vi "PrimaryAttackerRole_v2.vi"(7 "firstCall":bool=TRUE, 8 "error in (no error)":errorcluster, 10 "Game in":refnum<class "Game.lvclass">, 11 "ShootRole in":refnum<class "PrimaryAttackerRole_v2.lvclass">) -> (0 "error out":errorcluster, 1 "Game out":refnum<class "Game.lvclass">, 2 "Robot out":refnum<class "Robot.lvclass">, 3 "ShootRole out":refnum<class "PrimaryAttackerRole_v2.lvclass">)   [LabVIEW 2023, in "PrimaryAttackerRole_v2.lvclass"]
uses:
  PrimaryAttackerRole_v2.lvclass
  C:/Users/ebert/Documents/codes/SSL/repo/SSL_AI/Role_class/Role.lvclass
  Game_class/Game.lvclass
  Robot_class/Robot.lvclass
  Role_class/Role.lvclass/Role.ctl
  PrimaryAttacker_class/PrimaryAttackerRole_states.ctl
  PrimaryAttackerRole_v2.lvclass/PrimaryAttackerRole_v2.ctl
  Robot_class/tactics.ctl
  Robot_class/Robot.lvclass/Robot.ctl
  Tacticbook_class/Tacticbook.lvclass/Tacticbook.ctl
  Tacticbook_class/Read WaitPassTactic.vi
  Robot_class/Write tactic.vi
  Tacticbook_class/Read ShootTactic.vi
  Role_class/Read Tacticbook.vi
  Read Tactics.vi
  Role_class/Write Tacticbook.vi
  Write Tactics.vi
  Role_class/Write tactic_index.vi
  Role_class/Read RobotRef.vi
  Tacticbook_class/Tacticbook.lvclass
  Tactics/InterceptBallTactic_v2_class/InterceptBallTactic_v2.lvclass
  WaitPassTactic_class/WaitPassTactic.lvclass
  ShootTactic_class/ShootTactic.lvclass
  PrimaryAttacker_class/PrimaryAttackerRole.lvclass
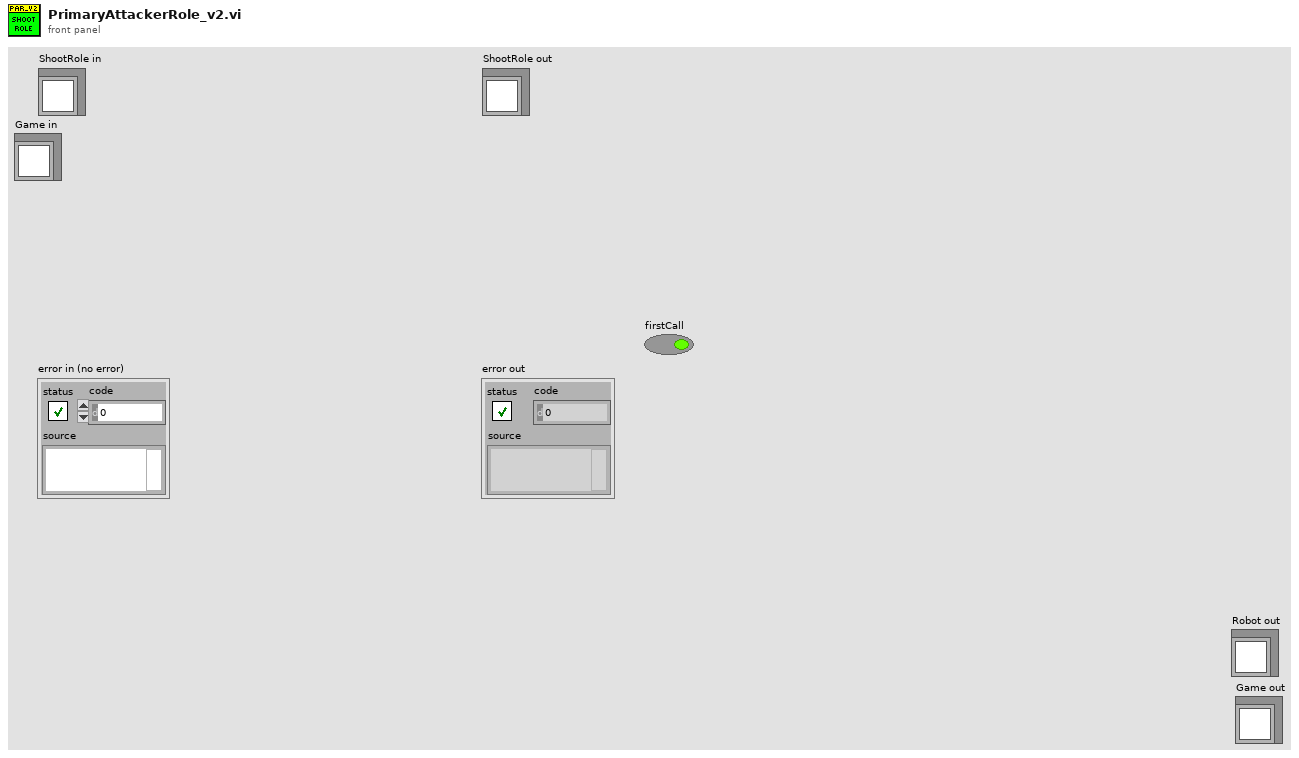
[diagram p1: front panel]
types:
  T1 = typedef "PrimaryAttackerRole.lvclass/PrimaryAttackerRole_states.ctl" = enum16{"Intercept", "PrepareShot", "Shoot", "Pass"}
  T2 = typedef "tactics.ctl" = enum16{"GoToBallPlacementPosition", "PlaceBall", "GoToBallPlacement", "5Robots", "BallPlacementEnemy", "ReceivePassInFuturePoint", "Roller", "PrepareRollToPassRollerGoTo", "PrepareRollToPassReceiverGoTo", "WaitRoll", "PositionToRoll", "PenaltyAttacker", "PassObserver", "PenaltyDefense", "TableReceiverTactic", "Test", "DefendGoal", "Marker", "FollowAttacker", "DefendArea", "Shoot", "AttackerAimGoal", "AttackerBallOutOfField", "AttackerBlock", "AttackerStop", "Duelist", "Halt", "ZigZag", "GoTo", "Timeout", "KickToBestRobot", "KickToPassReceiver", "PositionToReceivePass", "WaitPass", "Position", "Intercept", "PrepareShot", "Pass"}
  T3 = cluster{"InterceptBallTactic_v2":refnum<class "InterceptBallTactic_v2.lvclass">}
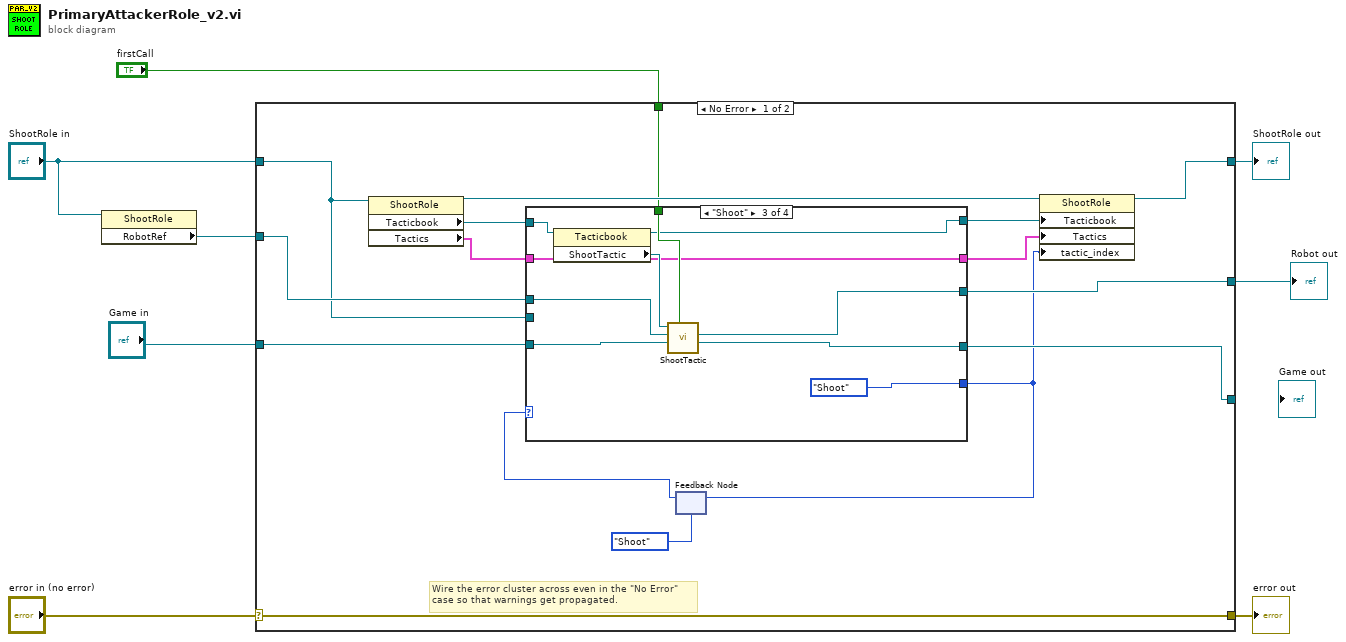
[diagram p0: block diagram]
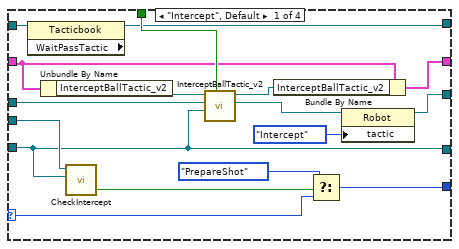
[diagram p2: hidden frame]
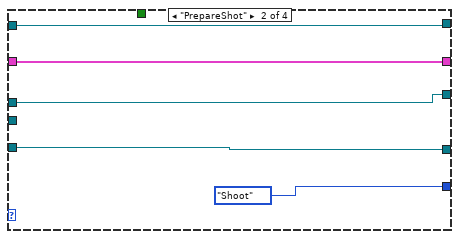
[diagram p3: hidden frame]
diagram:
  n1 = property class="ShootRole"(reference="ShootRole in") -> ("RobotRef"=w3:refnum<class "Robot.lvclass">)  [unwired: 1 in, 2 out]
  n2 = case shown="No Error" "error in (no error)" {
    selector: "error in (no error)" -> [w24 w65]
    tunnel: [w24 w65] -> w7
    tunnel: [w22 w64] -> w6
    tunnel: "ShootRole in" -> [w17 w64]
    tunnel: "Game in" -> [w20 w62]
    tunnel: w3 -> [w19 w63]
    tunnel: [w13 w63] -> w2
    tunnel: [w14 w62] -> _
    tunnel: "firstCall" -> [w21 _]
    frame No Error {
      # "Wire the error cluster across even in the \"No Error\"\ncase so that warnings get propagated."
      n3 = property class="ShootRole"(reference=w17) -> (reference out=w23:refnum<class "PrimaryAttackerRole_v2.lvclass">, "Tacticbook"=w11:refnum<class "Tacticbook.lvclass">, "Tactics"=w18:T3)  [unwired: 1 in, 1 out]
      n4 = feedback #1(PrimaryAttackerRole_states."Shoot" ("Enum")) -> (w15:T1)
      n5 = case shown="\"Shoot\"" w15 {
        selector: w15 -> [w32 _ _ w58]
        tunnel: [w41 PrimaryAttackerRole_states."Shoot" ("Enum") PrimaryAttackerRole_states."Shoot" ("Enum") w58] -> w10
        tunnel: w21 -> [w40 _ w54 _]
        tunnel: w20 -> [w26 w45 w52 w61]
        tunnel: w19 -> [w39 w46 w55 w59]
        tunnel: w18 -> [w30 w44 w50 w60]
        tunnel: w17 -> [w38 _ _ _]
        tunnel: [w26 w45 w51 w61] -> w14
        tunnel: [w31 w46 w49 w59] -> w13
        tunnel: [w29 w44 w50 w60] -> w12
        tunnel: w11 -> [w28 w42 w48 w57]
        tunnel: [w25 w42 w47 w57] -> w9
        frame "Intercept", Default {
          n6 = property class="Tacticbook" props=["WaitPassTactic"](reference=w28) -> (reference out=w25:refnum<class "Tacticbook.lvclass">)  [unwired: 1 in, 2 out]
          n7 = Unbundle By Name(w30) -> ("InterceptBallTactic_v2"=w37:refnum<class "InterceptBallTactic_v2.lvclass">)
          n8 = call-dynamic "CheckIntercept.vi"("Game"=w26, "object in"=w38) -> ("intercepted"=w36:bool)  [unwired: 7 in, 2 out]
          n9 = call-dynamic "InterceptBallTactic_v2.vi"("firstCall"=w40, "Game in"=w26, "Robot"=w39, "InterceptBallTactic_v2 in"=w37) -> ("Robot out"=w35:refnum<class "Robot.lvclass">, "InterceptBallTactic_v2 out"=w27:refnum<class "InterceptBallTactic_v2.lvclass">)  [unwired: 5 in, 1 out]
          n10 = Bundle By Name(cluster=w30, "InterceptBallTactic_v2"=w27) -> (w29:T3)
          n11 = Select(t=PrimaryAttackerRole_states."PrepareShot" ("Enum"), s=w36, f=w32) -> (s? t:f=w41:T1)
          n12 = property class="Robot"(reference=w35, "tactic"=tactics."Intercept") -> (reference out=w31:refnum<class "Robot.lvclass">)  [unwired: 1 in, 1 out]
        }
        frame "PrepareShot" {
        }
        frame "Shoot" {
          n13 = property class="Tacticbook"(reference=w48) -> (reference out=w47:refnum<class "Tacticbook.lvclass">, "ShootTactic"=w56:refnum<class "ShootTactic.lvclass">)  [unwired: 1 in, 1 out]
          n14 = call "ShootTactic.vi"("firstCall?"=w54, "Game in"=w52, "Robot"=w55, "ShootTactic in"=w56) -> ("Game out"=w51:refnum<class "Game.lvclass">, "Robot out"=w49:refnum<class "Robot.lvclass">)  [unwired: 4 in, 2 out]
        }
        frame "Pass" {
        }
      }
      n15 = feedback-in #1(w10) -> ()
      n16 = property class="ShootRole"(reference=w23, "Tacticbook"=w9, "Tactics"=w12, "tactic_index"=w10) -> (reference out=w22:refnum<class "PrimaryAttackerRole_v2.lvclass">)  [unwired: 1 in, 1 out]
    }
    frame Error {
    }
  }
  "error out" <- w7
  "ShootRole out" <- w6
  "Robot out" <- w2
